vi "lightsource-close.vi"(1 "VISA in":refnum<visa-resource-name>, 7 "NKT Input Cluster":T2={"Power Level"=5.0, "Feedback Level"=0.0, "Short Wavelength (nm)"=560, "Long Wavelength (nm)"=580, "UV Wavelength (nm)"=400, "Emission On/Off"=FALSE, "Power/Feedback Mode"=FALSE} {"UV Wavelength (nm)" min=350 max=480 step=1; "Long Wavelength (nm)" min=501 max=850 step=1; "Short Wavelength (nm)" min=400 max=560 step=1; "Feedback Level" min=0.0 max=90.0 step=0.1 format="%.1f%%"; "Power Level" min=5.0 max=100.0 step=0.1 format="%.1f%%"}) -> ()   [LabVIEW 2015]
panel:
  in  "PortParameters":T1={"OpenPort"=FALSE, "ClosePort"=FALSE, "Baudrate"=115200, "Wait"=50, "ReadWrite"=TRUE}
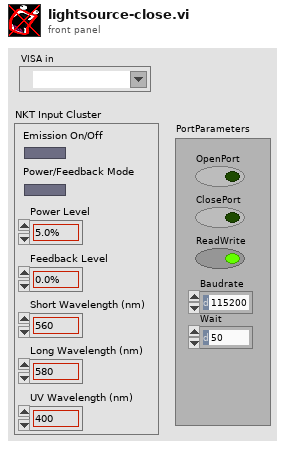
[diagram p1: front panel]
types:
  T1 = cluster{"OpenPort":bool, "ClosePort":bool, "Baudrate":i32, "Wait":u16, "ReadWrite":bool}
  T2 = cluster{"Power Level":dbl, "Feedback Level":dbl, "Short Wavelength (nm)":i32, "Long Wavelength (nm)":i32, "UV Wavelength (nm)":i32, "Emission On/Off":bool, "Power/Feedback Mode":bool}
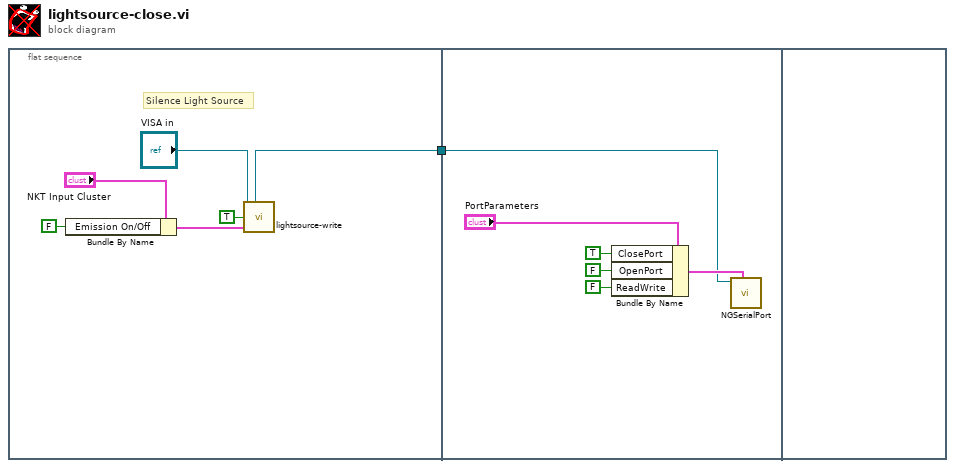
[diagram p0: block diagram]
diagram:
  n1 = flat-sequence {
    tunnel: [w3] -> w1
    tunnel: w1 -> [w8]
    frame #0 {
      # "Silence Light Source"
      n2 = Bundle By Name(cluster="NKT Input Cluster", "Emission On/Off"=FALSE) -> (w5:T2)
      n3 = call "lightsource-write.vi"("VISA in"="VISA in", "Init NKT?"=TRUE, "NKT Input Cluster"=w5) -> ("VISA out"=w3:refnum<visa-resource-name>)  [unwired: 3 in, 2 out]
    }
    frame #1 {
      n4 = Bundle By Name(cluster="PortParameters", "ClosePort"=TRUE, "OpenPort"=FALSE, "ReadWrite"=FALSE) -> (w9:T1)
      n5 = call "NGSerialPort.vi"("PortParameters"=w9, "VISA in"=w8) -> ()  [unwired: 7 in, 3 out]
    }
    frame #2 {
    }
  }
